vi "regex.vi"(7 "property_name":string, 8 "error_in":errorcluster, 10 "preregistration_data_content_in":string) -> (0 "error_out":errorcluster, 2 "preregistration_data_content_out":string, 4 "property_value":string, 6 "property_value_num":dbl)   [LabVIEW 2018]
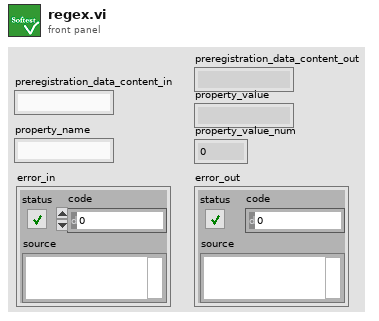
[diagram p1: front panel]
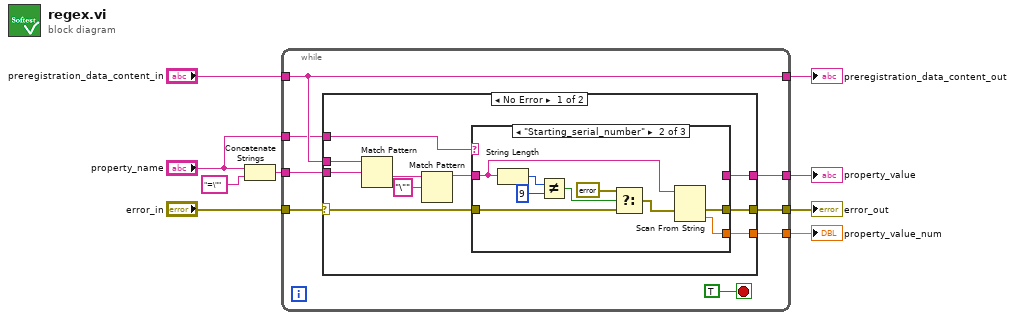
[diagram p0: block diagram]
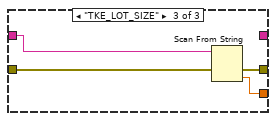
[diagram p3: hidden frame]
diagram:
  n1 = Concatenate Strings("property_name", "=\"" ("string")) -> (w4:string)
  n2 = while {
    tunnel: "preregistration_data_content_in" -> [w12]
    tunnel: w4 -> [w16]
    tunnel: [w17] -> w9
    tunnel: "error_in" -> [w14]
    tunnel: [w13] -> w6
    tunnel: [w12] -> w5
    tunnel: [w11] -> w2
    tunnel: "property_name" -> [w10]
    stop <- TRUE stop-if-true
    n3 = case shown="No Error" w14 {
      selector: w14 -> [w23 w43]
      tunnel: [w21 _] -> w17
      tunnel: w16 -> [w24 _]
      tunnel: [w20 w43] -> w13
      tunnel: w12 -> [w25 _]
      tunnel: [w19 _] -> w11
      tunnel: w10 -> [w18 _]
      frame No Error {
        n4 = Match Pattern(string=w25, regular expression=w24) -> (after substring=w26:string)  [unwired: 1 in, 3 out]
        n5 = Match Pattern(string=w26, regular expression="\"") -> (before substring=w22:string)  [unwired: 1 in, 3 out]
        n6 = case shown="\"Starting_serial_number\"" w18 {
          tunnel: w23 -> [w28 w35 w39]
          tunnel: w22 -> [w29 w31 w41]
          tunnel: [w29 _ _] -> w21
          tunnel: [w28 w32 w42] -> w20
          tunnel: [_ w30 w40] -> w19
          frame Default {
          }
          frame "Starting_serial_number" {
            n7 = String Length(string=w31) -> (length=w38:i32)
            n8 = Not Equal?(x=w38, y=9) -> (x != y?=w36:bool)
            n9 = Select(t=errorcluster {"status"=TRUE, "code"=0, "source"="Wrong serial number length"}, s=w36, f=w35) -> (s? t:f=w33:errorcluster)
            n10 = Scan From String(input string=w31, error in=w33) -> (error out=w32:errorcluster, output 1=w30:dbl)  [unwired: 3 in, 2 out]
          }
          frame "TKE_LOT_SIZE" {
            n11 = Scan From String(input string=w41, error in=w39) -> (error out=w42:errorcluster, output 1=w40:dbl)  [unwired: 3 in, 2 out]
          }
        }
      }
      frame Error {
      }
    }
  }
  "property_value" <- w9
  "error_out" <- w6
  "preregistration_data_content_out" <- w5
  "property_value_num" <- w2
